vi "车牌识别.vi"() -> ()   [LabVIEW 2013]
uses:
  <vilib>/vision/NI_Vision_Development_Module.lvlib
panel:
  in  "File Path *.abc":path=path "D:/车牌识别(精简版/T4.abc"
  out "输出簇":T1 {"Rotation" format="%.2f"; "Left" scale=0.0..1024.0; "Right" scale=0.0..1024.0}
  in  "Rectangle 2":T2
  in  "File  *.bmp":path
  in  "Rectangle":T1={"Left"=306, "Top"=214, "Right"=519, "Bottom"=287, "Rotation"=0.0} {"Rotation" format="%.2f"; "Left" scale=0.0..1024.0; "Right" scale=0.0..1024.0}
  out "String (OCR/OCV 1)":string
  out "Extarct":T3(plugin-control)
  out "Source":T3(plugin-control)
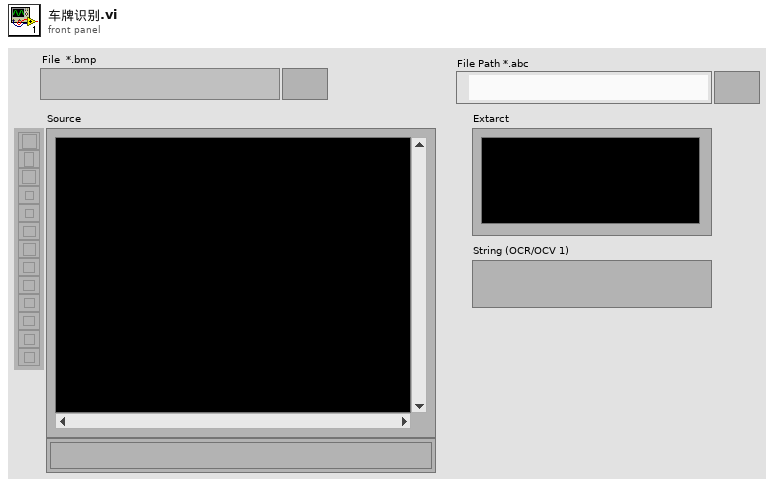
[diagram p1: front panel]
types:
  T1 = typedef "IMAQ Rectangle" = cluster{"Left":i32, "Top":i32, "Right":i32, "Bottom":i32, "Rotation":dbl}
  T2 = cluster{"Left":i32, "Top":i32, "Right":i32, "Bottom":i32}
  T3 = typedef "IMAQ Image.ctl" = refnum<image>
  T4 = typedef "Image Type" = u32
  T5 = cluster{"Threshold Data":cluster{"Method":enum16{"Fixed Range", "Uniform", "Linear", "Non Linear", "Local", "Color"}, "Looking for":u32, "Color Mode":u32, "Kernel Size":cluster{"Width":i32, "Height":i32}, "Ranges":cluster{"Min":i32, "Max":i32}[]}, "Reject Border":bool, "Number Of Erosions":i32, "Size & Spacing":cluster{"Segment Algorithm":u16, "Min Bounding Rect Width":i32, "Max Bounding Rect Width":i32, "Min Bounding Rect Height":i32, "Max Bounding Rect Height":i32, "Min Character Size":i32, "Max Character Size":i32, "Min Char Spacing":i32, "Max Horiz Element Spacing":i32, "Max Vert Element Spacing":i32, "Max Space Distance":i32}, "Read Options":cluster{"Read Strategy":i32, "Read Resolution":i32, "Scale Dependant":bool, "Aspect Ratio":i32, "Acceptance Level":i32, "Substitution Character":string, "MultiLine":bool}, "Valid Characters":cluster{"Pre-defined characters":i32, "User-defined characters":string}[], "Use Text Pattern":bool, "Orientation":u32, "# Lines Expected":u32, "Number of Blocks":i32}
  T6 = cluster{"Pixels ":cluster{"Start":cluster{"X":dbl, "Y":dbl}, "End":cluster{"X":dbl, "Y":dbl}}, "Real World":cluster{"Start":cluster{"X":dbl, "Y":dbl}, "End":cluster{"X":dbl, "Y":dbl}}}
  T7 = typedef "ROI Descriptor" = cluster{"Global Rectangle":i32[], "Contours":cluster{"ID":enum32{"External", "Internal"}, "Type":u32, "Coordinates":i32[]}[]}
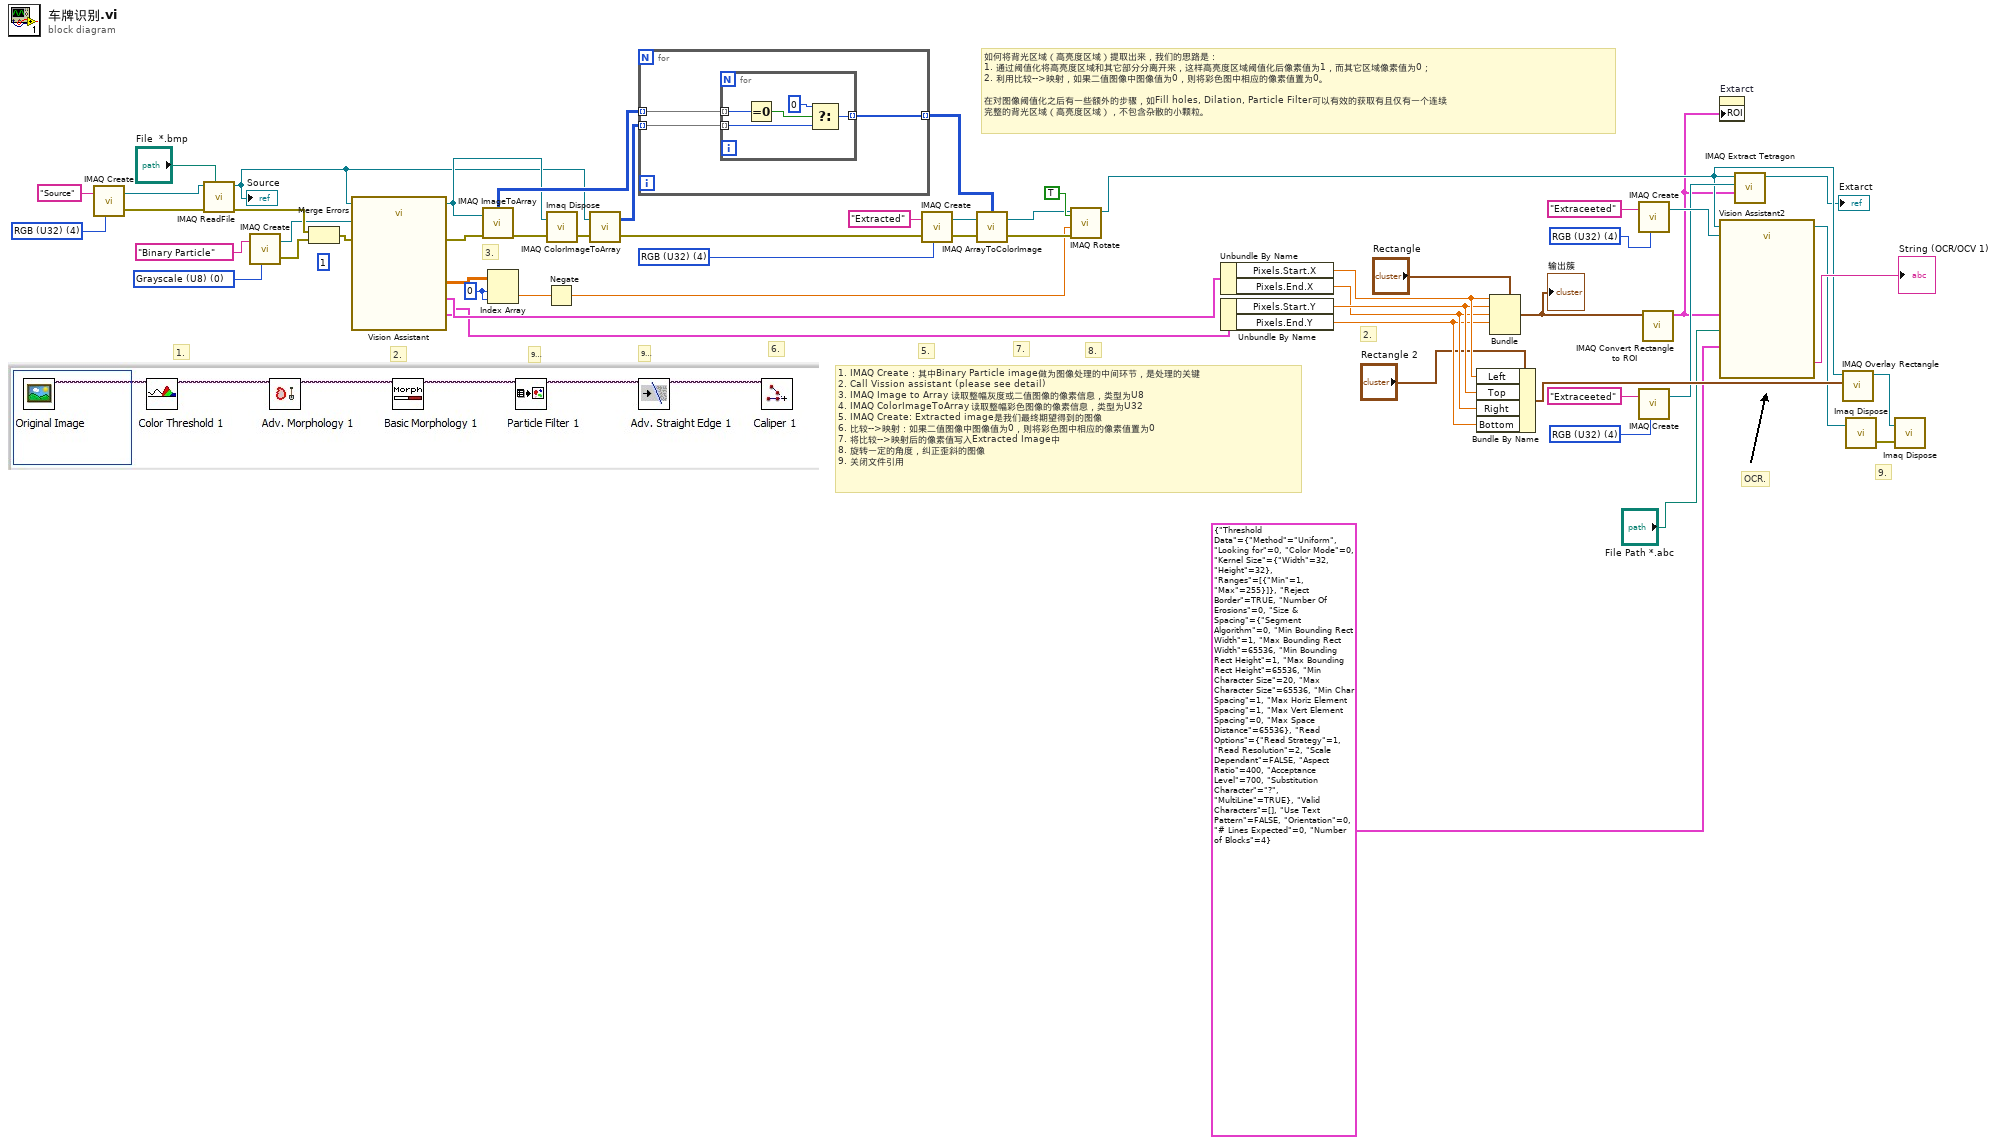
[diagram p0: block diagram]
diagram:
  w17 = T4 4 items=["Grayscale (U8)", "Grayscale (I16)", "Grayscale (SGL)", "Complex (CSG)", "RGB (U32)", "HSL (U32)", "RGB (U64)", "Grayscale (U16)"] ("Image Type")
  w20 = T4 4 items=["Grayscale (U8)", "Grayscale (I16)", "Grayscale (SGL)", "Complex (CSG)", "RGB (U32)", "HSL (U32)", "RGB (U64)", "Grayscale (U16)"] ("Image Type")
  (unwired) 1 ("Window Number (0...15)")
  w44 = 0 ("index (row)")
  w49 = T4 4 items=["Grayscale (U8)", "Grayscale (I16)", "Grayscale (SGL)", "Complex (CSG)", "RGB (U32)", "HSL (U32)", "RGB (U64)", "Grayscale (U16)"] ("Image Type")
  w52 = T4 0 items=["Grayscale (U8)", "Grayscale (I16)", "Grayscale (SGL)", "Complex (CSG)", "RGB (U32)", "HSL (U32)", "RGB (U64)", "Grayscale (U16)"] ("Image Type")
  w53 = T4 4 items=["Grayscale (U8)", "Grayscale (I16)", "Grayscale (SGL)", "Complex (CSG)", "RGB (U32)", "HSL (U32)", "RGB (U64)", "Grayscale (U16)"] ("Image Type")
  # "OCR."
  # "94"
  # "2."
  # "6."
  # "如何将背光区域（高亮度区域）提取出来，我们的思路是：\n1. 通过阈值化将高亮度区域和其它部分分离开来，这样高亮度区域阈值化后像素值为1，而其它区域像素值为0；\n2. 利用比较-->映射，如果二值图像中图像值为0，则将彩色图中相应的像素值置为0。\n\n在对图像阈值化之后有一些额外的步骤，如Fill holes, Dilation, Particle Filter可以有效的获取有且仅有一个连续\n完整的背光区域（高亮度区域），不包含杂散的小颗粒。"
  # "1. IMAQ Create：其中Binary Particle image做为图像处理的中间环节，是处理的关键\n2. Call Vission assistant (please see detail)\n3. IMAQ Image to Array 读取整幅灰度或二值图像的像素信息，类型为U8\n4. IMAQ ColorImageToArray 读取整幅彩色图像的像素信息，类型为U32\n5. IMAQ Create: Extracted image是我们最终期望得到的图像\n6. 比较-->映射：如果二值图像中图像值为0，则将彩色图中相应的像素值置为0\n7. 将比较-->映射后的像素值写入Extracted Image中\n8. 旋转一定的角度，纠正歪斜的图像\n9. 关闭文件引用"
  # "93"
  # "8."
  # "7."
  # "5."
  # "9."
  # "3."
  # "2."
  # "1."
  n1 = call "IMAQ Create"("Image Name"="Source", "Image Type"=w53) -> ("New Image"=w56:T3, "error out"=w54:errorcluster)  [unwired: 3 in]
  n2 = call "IMAQ ReadFile"("File Path"="File  *.bmp", "error in (no error)"=w54, "Image"=w56) -> ("error out"=w38:errorcluster, "Image Out"=w10:T3)  [unwired: 4 in, 3 out]
  "Source" <- w10
  n3 = call "IMAQ Create"("Image Name"="Binary Particle", "Image Type"=w52) -> ("New Image"=w29:T3, "error out"=w28:errorcluster)  [unwired: 3 in]
  n4 = Merge Errors(w38, w28) -> (w37:errorcluster)
  n5 = call "Vision Assistant"("Image In"=w10, "Image Dst"=w29, "error in"=w37) -> ("Image Out"=w32:T3, "Caliper Results (Caliper 1)"=w45:sgl[][], "Clamp Points (Max Clamp 1)"=w4:T6, "Clamp Points (Max Clamp 2)"=w3:T6, "error out"=w39:errorcluster)  [unwired: 20 in]
  n6 = call "IMAQ ImageToArray"("error in (no error)"=w39, "Image"=w32) -> ("error out"=w34:errorcluster, "Image Pixels (U8)"=w47:u8[][])  [unwired: 2 in, 3 out]
  n7 = Index Array(array=w45, index (row)=w44, index (col)=w44) -> (element=w43:sgl)
  n8 = Negate(x=w43) -> (-x=w2:sgl)
  n9 = call "Imaq Dispose"("Image"=w32, "error in (no error)"=w34) -> ("error out"=w33:errorcluster)  [unwired: 4 in]
  n10 = call "IMAQ ColorImageToArray"("Image"=w10, "error in (no error)"=w33) -> ("Image Pixels (U32)"=w48:u32[][], "error out"=w36:errorcluster)  [unwired: 2 in, 1 out]
  n11 = for {
    tunnel: w48 -> [w59] mode=indexing
    tunnel: w47 -> [w58] mode=indexing
    tunnel: [w57] -> w15 mode=indexing
    n12 = for {
      tunnel: w59 -> [w62] mode=indexing
      tunnel: w58 -> [w64] mode=indexing
      tunnel: [w60] -> w57 mode=indexing
      n13 = Equal To 0?(x=w64) -> (x = 0?=w63:bool)
      n14 = Select(t=u32 0, s=w63, f=w62) -> (s? t:f=w60:u32)
    }
  }
  n15 = call "IMAQ Create"("Image Name"="Extracted", "Image Type"=w49, "error in (no error)"=w36) -> ("New Image"=w40:T3, "error out"=w35:errorcluster)  [unwired: 2 in]
  n16 = call "IMAQ ArrayToColorImage"("Image Pixels (U32)"=w15, "Image"=w40, "error in (no error)"=w35) -> ("Image Out"=w41:T3, "error out"=w42:errorcluster)  [unwired: 2 in]
  n17 = call "IMAQ Rotate"("Maintain Size"=TRUE, "error in (no error)"=w42, "Angle (degrees)"=w2, "Image Src"=w41) -> ("Image Dst Out"=w8:T3)  [unwired: 4 in, 3 out]
  n18 = Unbundle By Name(w4) -> ("Pixels.Start.X"=w14:dbl, "Pixels.End.X"=w12:dbl)
  n19 = Unbundle By Name(w3) -> ("Pixels.Start.Y"=w13:dbl, "Pixels.End.Y"=w11:dbl)
  n20 = Bundle By Name(cluster="Rectangle 2", "Left"=w14, "Top"=w13, "Right"=w12, "Bottom"=w11) -> (w27:T2)
  n21 = Bundle(cluster="Rectangle", "Left"=w14, "Top"=w13, "Right"=w12, "Bottom"=w11) -> (w25:T1)  [unwired: 1 in]
  "输出簇" <- w25
  n22 = call "IMAQ Create"("Image Name"="Extraceeted", "Image Type"=w20) -> ("New Image"=w19:T3)  [unwired: 3 in, 1 out]
  n23 = call "IMAQ Create"("Image Name"="Extraceeted", "Image Type"=w17) -> ("New Image"=w9:T3)  [unwired: 3 in, 1 out]
  n24 = call "IMAQ Convert Rectangle to ROI"("Rectangle"=w25) -> ("ROI Descriptor"=w5:T7)  [unwired: 8 in, 1 out]
  n25 = property on="Extarct" class="ImageControl"("ROI"=w5) -> ()  [unwired: 2 in, 2 out]
  n26 = call "Vision Assistant2"("Image In"=w8, "Image Dst"=w19, "ROI Descriptor (OCR/OCV 1)"=w5, "File Path (OCR/OCV 1)"="File Path *.abc", "Parameters (OCR/OCV 1)"=T5 {"Threshold Data"={"Method"=enum."Uniform", "Looking for"=0, "Color Mode"=0, "Kernel Size"={"Width"=32, "Height"=32}, "Ranges"=[{"Min"=1, "Max"=255}]}, "Reject Border"=TRUE, "Number Of Erosions"=0, "Size & Spacing"={"Segment Algorithm"=0, "Min Bounding Rect Width"=1, "Max Bounding Rect Width"=65536, "Min Bounding Rect Height"=1, "Max Bounding Rect Height"=65536, "Min Character Size"=20, "Max Character Size"=65536, "Min Char Spacing"=1, "Max Horiz Element Spacing"=1, "Max Vert Element Spacing"=0, "Max Space Distance"=65536}, "Read Options"={"Read Strategy"=1, "Read Resolution"=2, "Scale Dependant"=FALSE, "Aspect Ratio"=400, "Acceptance Level"=700, "Substitution Character"="?", "MultiLine"=TRUE}, "Valid Characters"=[], "Use Text Pattern"=FALSE, "Orientation"=0, "# Lines Expected"=0, "Number of Blocks"=4}) -> ("Image Out"=w22:T3, "String (OCR/OCV 1)"=→"String (OCR/OCV 1)":string)  [unwired: 20 in, 1 out]
  n27 = call-poly "IMAQ Extract Tetragon"("ROI Descriptor"=w5, "Image Dst"=w9, "Image Src"=w8) -> ("Image Dst Out"=→"Extarct":T3)  [unwired: 7 in, 1 out]
  n28 = call "IMAQ Overlay Rectangle"("Rectangle"=w27, "Image"=w8) -> ("Image Out"=w18:T3)  [unwired: 8 in, 1 out]
  n29 = call "Imaq Dispose"("Image"=w22) -> ("error out"=w31:errorcluster)  [unwired: 5 in]
  n30 = call "Imaq Dispose"("Image"=w18, "error in (no error)"=w31) -> ()  [unwired: 4 in, 1 out]
